vi "Set Report Margins.vi"(0 "report in":refnum<class "NI_Excel.lvclass">, 5 "margins (1.00)":T1={"top"=1.0, "left"=1.0, "right"=1.0, "bottom"=1.0} {"right" format="%.2f"; "bottom" format="%.2f"; "top" format="%.2f"; "left" format="%.2f"}, 9 "measurement system (default)":u16(ring) items=["Default", "US", "Metric"], 11 "error in (no error)":errorcluster) -> (4 "report out":refnum<class "NI_Excel.lvclass">, 10 "page width (Word)":sgl format="%.2f", 15 "error out":errorcluster)   [LabVIEW 2015, in "NI_Excel.lvclass"]
doc: "Sets the margins of the specified report."
uses:
  <vilib>/Utility/NIReport.llb/Excel/NI_Excel.lvclass
  <vilib>/Utility/NIReport.llb/Excel/NI_Excel.lvclass/NI_Excel.ctl
  <vilib>/addons/_office/NI_ReportGenerationToolkit.lvlib
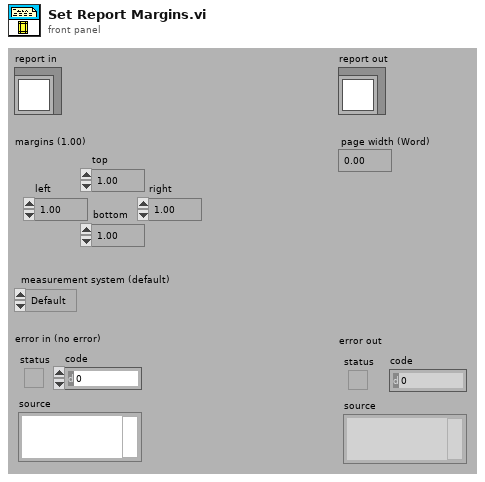
[diagram p1: front panel]
types:
  T1 = cluster{"top":dbl, "left":dbl, "right":dbl, "bottom":dbl}
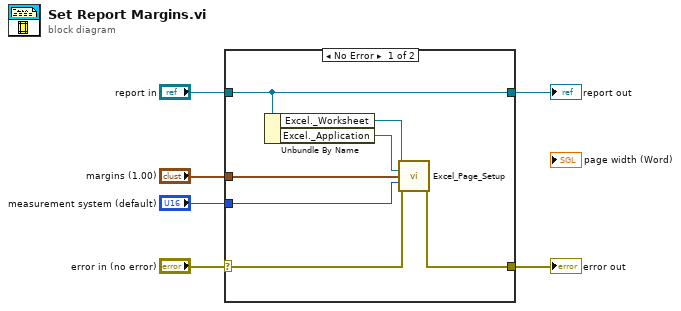
[diagram p0: block diagram]
diagram:
  n1 = case shown="No Error" "error in (no error)" {
    selector: "error in (no error)" -> [w10 w15]
    tunnel: [w9 w15] -> w5
    tunnel: [w11 w14] -> w3
    tunnel: "report in" -> [w11 w14]
    tunnel: "margins (1.00)" -> [w8 _]
    tunnel: "measurement system (default)" -> [w7 _]
    frame No Error {
      n2 = Unbundle By Name(w11) -> ("Excel._Worksheet"=w12:refnum<k7>, "Excel._Application"=w13:refnum<k7>)
      n3 = call <vilib>:"Excel_Page_Setup.vi"("Excel._Worksheet"=w12, "Excel._Application"=w13, "margins (1.00)"=w8, "measurement system (Default)"=w7, "error in (no error)"=w10) -> ("error out"=w9:errorcluster)  [unwired: 10 out]
    }
    frame Error {
    }
  }
  "error out" <- w5
  "report out" <- w3
